vi "microFPGA_analog_input_addr_46_ctrl.vi"(0 "VISA resource name":refnum<visa-resource-name>, 1 "analog readout channel":u16(ring)=3 items=["channel No 0", "channel No 1", "channel No 2", "channel No 3", "channel No 4", "channel No 5", "channel No 6", "channel No 7"], 11 "error in (no error)":errorcluster) -> (4 "VISA resource name 2":refnum<visa-resource-name>, 6 "analog value read":i32, 10 "abort_wrong_input":bool, 15 "error out":errorcluster)   [LabVIEW 2021]
panel:
  out "mode read string answer":string
  out "mode read string":string
  out "mode write string":string
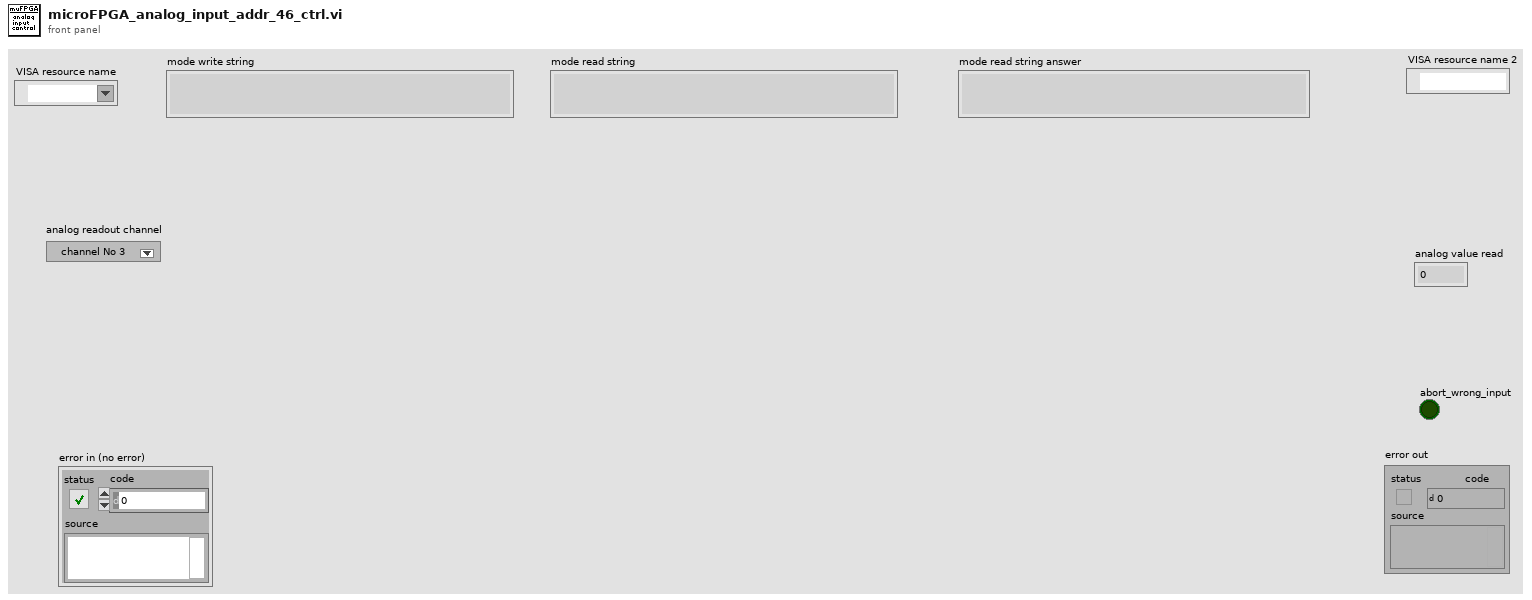
[diagram p1: front panel]
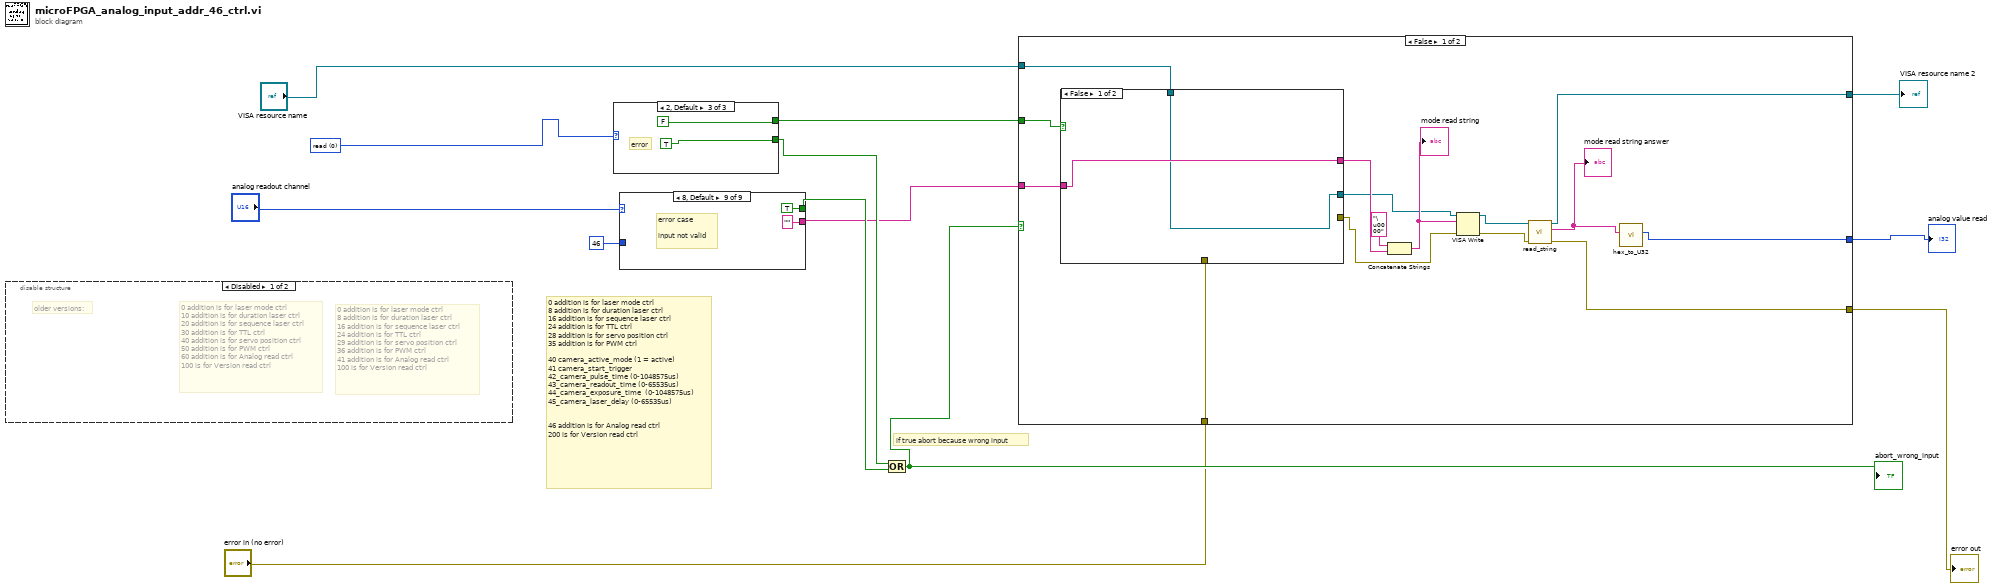
[diagram p0: block diagram]
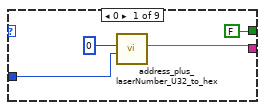
[diagram p3: hidden frame]
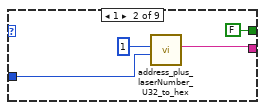
[diagram p4: hidden frame]
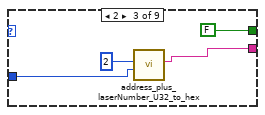
[diagram p5: hidden frame]
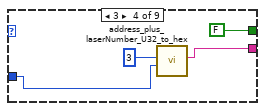
[diagram p6: hidden frame]
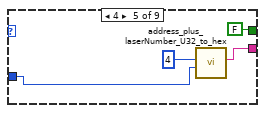
[diagram p7: hidden frame]
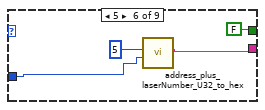
[diagram p8: hidden frame]
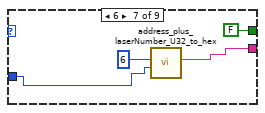
[diagram p9: hidden frame]
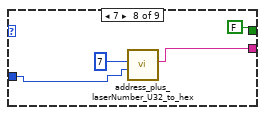
[diagram p10: hidden frame]
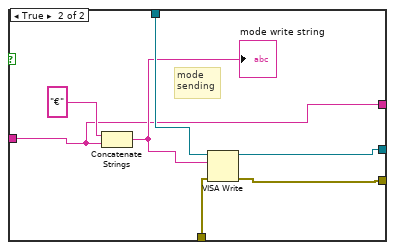
[diagram p11: hidden frame]
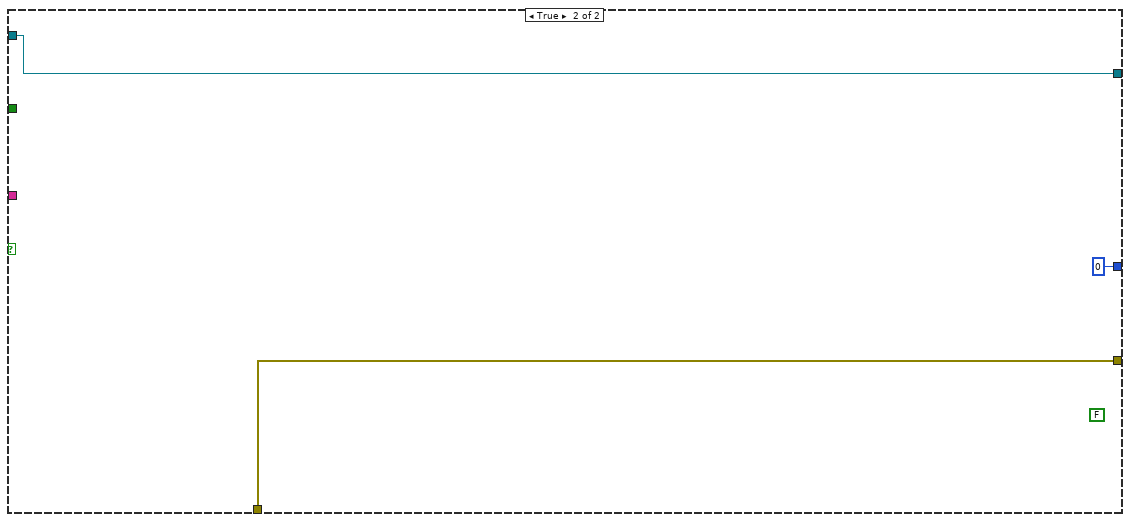
[diagram p12: hidden frame]
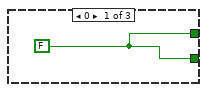
[diagram p13: hidden frame]
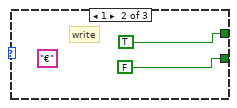
[diagram p14: hidden frame]
diagram:
  w12 = u16 0 items=["read", "write"] ("write or read")
  # "0 addition is for laser mode ctrl\n8 addition is for duration laser ctrl\n16 addition is for sequence laser ctrl\n24 addition is for TTL ctrl\n28 addition is for servo position ctrl\n35 addition is for PWM ctrl\n\n40 camera_active_mode (1 = active) \n41 camera_start_trigger\n42_camera_pulse_time (0-1048575us)\n43_camera_readout_time (0-65535us)\n44_camera_exposure_time  (0-1048575us)\n45_camera_laser_delay (0-65535us)\n\n\n46 addition is for Analog read ctrl\n200 is for Version read ctrl"
  # "if true abort because wrong input"
  n1 = disable-structure shown="Disabled" {
    frame Disabled {
      # "older versions:"
      # "0 addition is for laser mode ctrl\n8 addition is for duration laser ctrl\n16 addition is for sequence laser ctrl\n24 addition is for TTL ctrl\n29 addition is for servo position ctrl\n36 addition is for PWM ctrl\n41 addition is for Analog read ctrl\n100 is for Version read ctrl"
      # "0 addition is for laser mode ctrl\n10 addition is for duration laser ctrl\n20 addition is for sequence laser ctrl\n30 addition is for TTL ctrl\n40 addition is for servo position ctrl\n50 addition is for PWM ctrl\n60 addition is for Analog read ctrl\n100 is for Version read ctrl"
    }
    frame Enabled {
    }
  }
  n2 = case shown="2, Default" w12 {
    tunnel: [w14 TRUE FALSE] -> w11
    tunnel: [w14 FALSE TRUE] -> w10
    frame 0 {
      w14 = FALSE
    }
    frame 1 {
      (unwired) "€" ("hex")
      # "write"
    }
    frame 2, Default {
      # "error"
    }
  }
  n3 = case shown="8, Default" "analog readout channel" {
    tunnel: [w20 w24 w28 w32 w36 w40 w44 w47 "" ("string 5")] -> w2
    tunnel: [FALSE FALSE FALSE FALSE FALSE FALSE FALSE FALSE TRUE] -> w3
    tunnel: u32 46 ("adress offset") -> [w19 w23 w27 w31 w35 w39 w43 w48 _]
    frame 0 {
      n4 = call "address_plus_laserNumber_U32_to_hex.vi"("adress offset"=w19, "y 3"=u32 0) -> ("string 5"=w20:string)  [unwired: 8 in]
    }
    frame 1 {
      n5 = call "address_plus_laserNumber_U32_to_hex.vi"("adress offset"=w23, "y 3"=u32 1) -> ("string 5"=w24:string)  [unwired: 8 in]
    }
    frame 2 {
      n6 = call "address_plus_laserNumber_U32_to_hex.vi"("adress offset"=w27, "y 3"=u32 2) -> ("string 5"=w28:string)  [unwired: 8 in]
    }
    frame 3 {
      n7 = call "address_plus_laserNumber_U32_to_hex.vi"("adress offset"=w31, "y 3"=u32 3) -> ("string 5"=w32:string)  [unwired: 8 in]
    }
    frame 4 {
      n8 = call "address_plus_laserNumber_U32_to_hex.vi"("adress offset"=w35, "y 3"=u32 4) -> ("string 5"=w36:string)  [unwired: 8 in]
    }
    frame 5 {
      n9 = call "address_plus_laserNumber_U32_to_hex.vi"("adress offset"=w39, "y 3"=u32 5) -> ("string 5"=w40:string)  [unwired: 8 in]
    }
    frame 6 {
      n10 = call "address_plus_laserNumber_U32_to_hex.vi"("adress offset"=w43, "y 3"=u32 6) -> ("string 5"=w44:string)  [unwired: 8 in]
    }
    frame 7 {
      n11 = call "address_plus_laserNumber_U32_to_hex.vi"("adress offset"=w48, "y 3"=u32 7) -> ("string 5"=w47:string)  [unwired: 8 in]
    }
    frame 8, Default {
      # "error case\n\ninput not valid"
    }
  }
  n12 = Compound Arithmetic op=OR(w10, w3) -> (w9:bool)
  "abort_wrong_input" <- w9
  n13 = case shown="False" w9 {
    tunnel: "VISA resource name" -> [w67 w78]
    tunnel: w2 -> [w64 _]
    tunnel: w11 -> [w58 _]
    tunnel: [w56 u32 0 ("U32")] -> w1
    tunnel: [w55 w78] -> w8
    tunnel: "error in (no error)" -> [w54 w77]
    tunnel: [w53 w77] -> w6
    frame False {
      n14 = case shown="False" w58 {
        tunnel: w64 -> [w69 w73]
        tunnel: w67 -> [w68 w75]
        tunnel: [w69 w73] -> w65
        tunnel: [w68 w72] -> w60
        tunnel: [_ w71] -> w59
        tunnel: w54 -> [_ w70]
        frame False {
        }
        frame True {
          # "mode \nsending"
          n15 = Concatenate Strings("€" ("string"), w73) -> (w74:string)
          "mode write string" <- w74
          n16 = VISA Write(VISA resource name=w75, write buffer=w74, error in (no error)=w70) -> (VISA resource name out=w72:refnum<visa-resource-name>, error out=w71:errorcluster)  [unwired: 1 out]
        }
      }
      n17 = Concatenate Strings("\u0000" ("string"), w65) -> (w63:string)
      "mode read string" <- w63
      n18 = VISA Write(VISA resource name=w60, write buffer=w63, error in (no error)=w59) -> (VISA resource name out=w62:refnum<visa-resource-name>, error out=w61:errorcluster)  [unwired: 1 out]
      n19 = call "read_string.vi"("error in (no error)"=w61, "VISA resource name 2"=w62) -> ("error out"=w53:errorcluster, "read buffer"=w57:string, "VISA resource name"=w55:refnum<visa-resource-name>)  [unwired: 7 in]
      "mode read string answer" <- w57
      n20 = call "hex_to_U32.vi"("hex"=w57) -> ("U32"=w56:u32)  [unwired: 9 in]
    }
    frame True {
      (unwired) FALSE
    }
  }
  "VISA resource name 2" <- w8
  "error out" <- w6
  "analog value read" <- w1
